vi "Clean Up.vi"(8 "error in":errorcluster, 10 "Show":bool, 11 "Report Viewer in":refnum<class "Report Viewer.lvclass">) -> (0 "error out":errorcluster, 3 "Report Viewer out":refnum<class "Report Viewer.lvclass">)   [LabVIEW 2019, in "Report Viewer.lvlib" / "Report Viewer.lvclass"]
uses:
  Library/Report Viewer.lvclass
  Library/Report Viewer.lvclass/Report Viewer.ctl
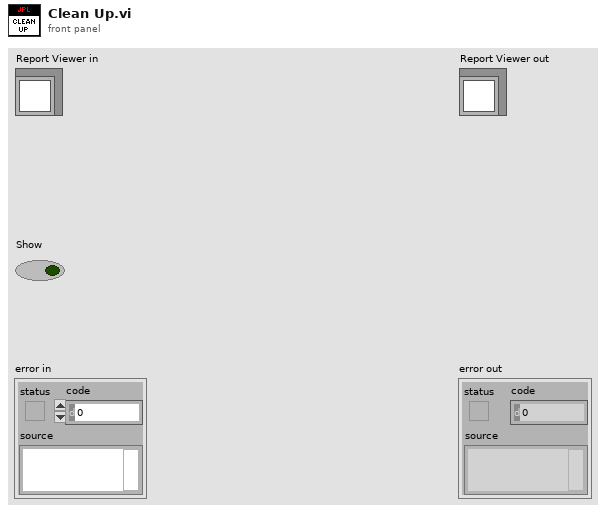
[diagram p1: front panel]
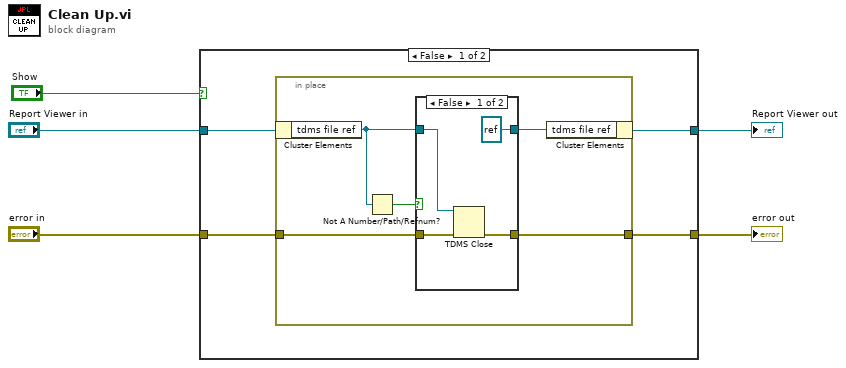
[diagram p0: block diagram]
diagram:
  n1 = case shown="False" "Show" {
    tunnel: "Report Viewer in" -> [w9 w22]
    tunnel: [w8 w22] -> w3
    tunnel: [w7 w21] -> w2
    tunnel: "error in" -> [w6 w21]
    frame False {
      n2 = in-place {
        in-place-border: [w11] -> w7
        in-place-border: w6 -> [w10]
        n3 = in-place-cluster #1(w9) -> ("tdms file ref"=w13:refnum<k34>)
        n4 = Not A Number/Path/Refnum?(number/path/refnum=w13) -> (NaN/Path/Refnum?=w14:bool)
        n5 = case shown="False" w14 {
          tunnel: w13 -> [w18 w20]
          tunnel: [refnum<k34> refnum ("tdms file ref") w20] -> w12
          tunnel: [w16 w19] -> w11
          tunnel: w10 -> [w15 w19]
          frame False {
            n6 = TDMS Close(8:w15, 11:w18) -> (0:w16:errorcluster)  [unwired: 1 out]
          }
          frame True {
          }
        }
        n7 = in-place-cluster #1("tdms file ref"=w12) -> (w8:refnum<class "Report Viewer.lvclass">)
      }
    }
    frame True {
    }
  }
  "error out" <- w2
  "Report Viewer out" <- w3
